vi "Format to Bold.vi"(8 "Adjust Height?":bool, 9 "String Value":string, 10 "String Ref":refnum<vi>) -> ()   [LabVIEW 2019, in "Panther Dashboard.lvlib"]
uses:
  Panther Dashboard.lvlib
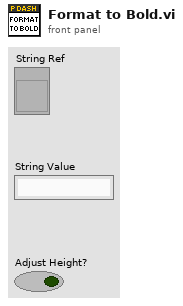
[diagram p1: front panel]
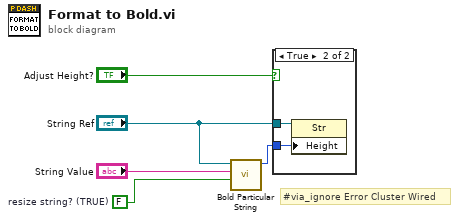
[diagram p0: block diagram]
diagram:
  w5 = FALSE  # resize string? (TRUE)
  # "#via_ignore Error Cluster Wired"
  n1 = call <vilib>:"Bold Particular String.vi"("resize string? (TRUE)"=w5, "text to display"="String Value", "string refnum"="String Ref") -> ("string control height"=w4:u32)  [unwired: 7 in, 1 out]
  n2 = case shown="True" "Adjust Height?" {
    tunnel: w4 -> [_ w7]
    tunnel: "String Ref" -> [_ w6]
    frame False {
    }
    frame True {
      n3 = property on="Property Node" class="Str"(reference=w6, "Height"=w7) -> ()  [unwired: 1 in, 2 out]
    }
  }
